vi "shutdown background process.vi"(8 "error in":errorcluster, 11 "async data":T1) -> (0 "error out":errorcluster, 3 "module out":refnum<class "TBM module execution interface.lvclass">)   [LabVIEW 2013, in "Standard Engine Runtime.lvclass"]
uses:
  Standard Engine Runtime.lvclass
  <vilib>/NI/Tag Bus Module Framework/runtime/TBM module execution interface.lvclass
  async command notification.ctl
  <vilib>/NI/Tag Bus/table/data table.ctl
  <vilib>/NI/Tag Bus/table/data table.lvlib
  <vilib>/NI/Tag Bus Module Framework/runtime/execution settings.ctl
  asynchronous process data.ctl
  <vilib>/NI/Tag Bus Module Framework/runtime/error classification.ctl
  async error info.ctl
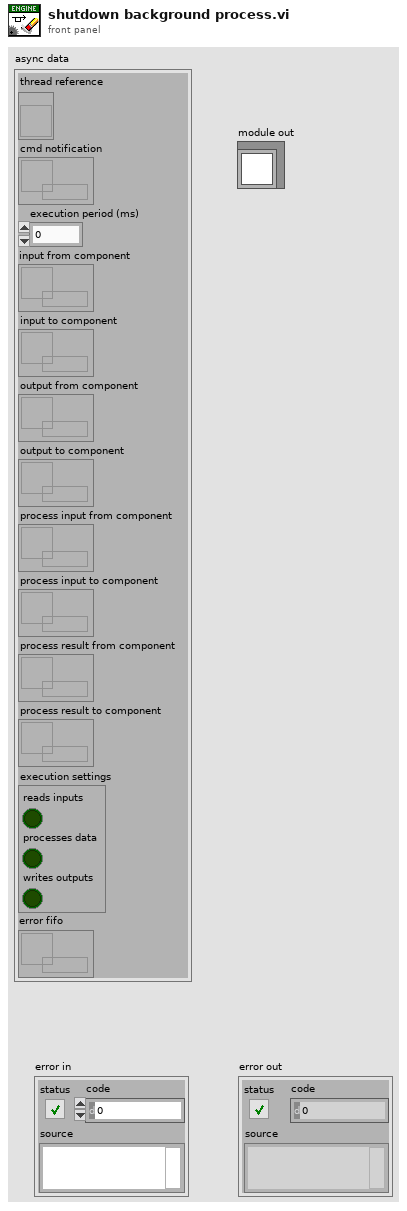
[diagram p1: front panel]
types:
  T1 = typedef "Standard Engine Runtime.lvclass/asynchronous process data.ctl" = cluster{"thread reference":refnum<vi>, "cmd notification":refnum<k33>, "execution period (ms)":i32, "input from component":refnum<queue>, "input to component":refnum<queue>, "output from component":refnum<queue>, "output to component":refnum<queue>, "process input from component":refnum<queue>, "process input to component":refnum<queue>, "process result from component":refnum<queue>, "process result to component":refnum<queue>, "execution settings":T2, "error fifo":refnum<k33>}
  T2 = typedef "TBM module execution interface.lvclass/execution settings.ctl" = cluster{"reads inputs":bool, "processes data":bool, "writes outputs":bool}
  T3 = typedef "Standard Engine Runtime.lvclass/async command notification.ctl" = enum16{"stop", "safe state", "recover"}
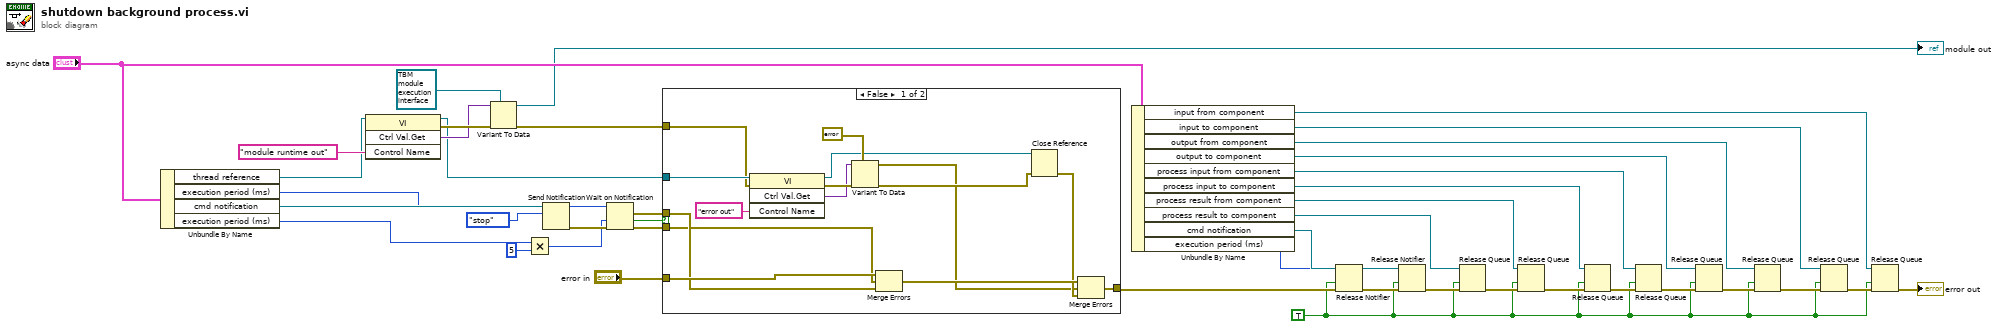
[diagram p0: block diagram]
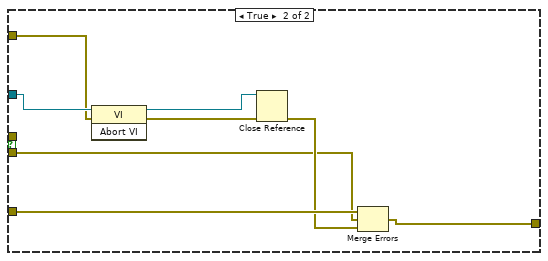
[diagram p2: hidden frame]
diagram:
  w2 = TRUE ("force destroy? (F)")
  n1 = Unbundle By Name("async data") -> ("thread reference"=w5:refnum<vi>, "execution period (ms)"=w41:i32, "cmd notification"=w42:refnum<k33>, "execution period (ms)"=w16:i32)
  n2 = invoke class="VI" method="Ctrl Val.Get"(reference=w5, "Control Name"="module runtime out") -> (reference out=w6:refnum<vi>, error out=w9:errorcluster, "Get Control Value Variant"=w7:variant)  [unwired: 2 in, 1 out]
  n3 = Variant To Data(error in=w9, type=refnum<class "TBM module execution interface.lvclass"> refnum ("module runtime out"), Variant=w7) -> (data=→"module out":refnum<class "TBM module execution interface.lvclass">, error out=w4:errorcluster)
  n4 = Multiply(x=w16, y=5) -> (x*y=w14:i32)
  n5 = Send Notification(notification=async_command_notification."stop", notifier=w42) -> (error out=w40:errorcluster)  [unwired: 1 in, 1 out]
  n6 = Wait on Notification(notifier=w41, timeout in ms (-1)=w14, error in (no error)=w40) -> (notification=w37:errorcluster, timed out?=w39:bool, error out=w38:errorcluster)  [unwired: 1 in, 1 out]
  n7 = case shown="False" w39 {
    tunnel: w38 -> [w43 w58]
    tunnel: w37 -> [w56 _]
    tunnel: "error in" -> [w57 w65]
    tunnel: [w53 w63] -> w36
    tunnel: w6 -> [w52 w61]
    tunnel: w4 -> [w44 w59]
    frame False {
      n8 = invoke class="VI" method="Ctrl Val.Get"(reference=w52, error in=w44, "Control Name"="error out") -> (reference out=w47:refnum<vi>, error out=w50:errorcluster, "Get Control Value Variant"=w49:variant)  [unwired: 1 in, 1 out]
      n9 = Variant To Data(error in=w50, type=errorcluster {"status"=FALSE, "code"=0, "source"=""} ("error constant"), Variant=w49) -> (data=w45:errorcluster, error out=w46:errorcluster)
      n10 = Merge Errors(w57, w43, w56) -> (w55:errorcluster)
      n11 = Close Reference(reference=w47, error in (no error)=w46) -> (error out=w54:errorcluster)
      n12 = Merge Errors(w55, w45, w54) -> (w53:errorcluster)
    }
    frame True {
      n13 = invoke class="VI" method="Abort VI"(reference=w61, error in=w59) -> (reference out=w60:refnum<vi>, error out=w62:errorcluster)  [unwired: 1 in, 1 out]
      n14 = Close Reference(reference=w60, error in (no error)=w62) -> (error out=w64:errorcluster)
      n15 = Merge Errors(w65, w58, w64) -> (w63:errorcluster)
    }
  }
  n16 = Unbundle By Name("async data") -> ("input from component"=w17:refnum<queue>, "input to component"=w18:refnum<queue>, "output from component"=w19:refnum<queue>, "output to component"=w20:refnum<queue>, "process input from component"=w30:refnum<queue>, "process input to component"=w29:refnum<queue>, "process result from component"=w28:refnum<queue>, "process result to component"=w27:refnum<queue>, "cmd notification"=w26:refnum<k33>, "execution period (ms)"=w25:i32)
  n17 = Release Notifier(notifier=w25, force destroy? (F)=w2, error in (no error)=w36) -> (error out=w35:errorcluster)  [unwired: 2 out]
  n18 = Release Notifier(notifier=w26, force destroy? (F)=w2, error in (no error)=w35) -> (error out=w31:errorcluster)  [unwired: 2 out]
  n19 = Release Queue(queue=w27, force destroy? (F)=w2, error in (no error)=w31) -> (error out=w32:errorcluster)  [unwired: 2 out]
  n20 = Release Queue(queue=w28, force destroy? (F)=w2, error in (no error)=w32) -> (error out=w33:errorcluster)  [unwired: 2 out]
  n21 = Release Queue(queue=w29, force destroy? (F)=w2, error in (no error)=w33) -> (error out=w34:errorcluster)  [unwired: 2 out]
  n22 = Release Queue(queue=w30, force destroy? (F)=w2, error in (no error)=w34) -> (error out=w21:errorcluster)  [unwired: 2 out]
  n23 = Release Queue(queue=w20, force destroy? (F)=w2, error in (no error)=w21) -> (error out=w24:errorcluster)  [unwired: 2 out]
  n24 = Release Queue(queue=w19, force destroy? (F)=w2, error in (no error)=w24) -> (error out=w23:errorcluster)  [unwired: 2 out]
  n25 = Release Queue(queue=w18, force destroy? (F)=w2, error in (no error)=w23) -> (error out=w22:errorcluster)  [unwired: 2 out]
  n26 = Release Queue(queue=w17, force destroy? (F)=w2, error in (no error)=w22) -> (error out=→"error out":errorcluster)  [unwired: 2 out]
